vi "GlobalCCDMaxDim.vi"() -> ()   [LabVIEW 2010]
panel:
  in  "CCD Max Y":u32
  in  "CCD Max X":u32
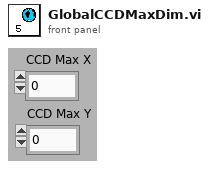
[diagram p1: front panel]
diagram:
